vi "test_scope.vi"() -> ()   [LabVIEW 2009]
uses:
  <instrlib>/Agilent 8000 Series/Agilent 8000 Series.lvlib
panel:
  out "bucle time":u32
  in  "stop while":bool
  in  "Boolean ini":bool
  in  "write buffer ini":string
  in  "byte count 2":u32
  out "return count 4":u32
  out "return count 3":u32
  out "return count 2":u32
  out "return count":u32
  in  "byte count":u32
  out "Numeric":i32
  out "read buffer":string
  out "error out":errorcluster
  in  "VISA resource name":refnum<visa-resource-name>
  in  "stop":bool
  in  "write buffer":string
  out "x-y":u32
  in  "Boolean":bool
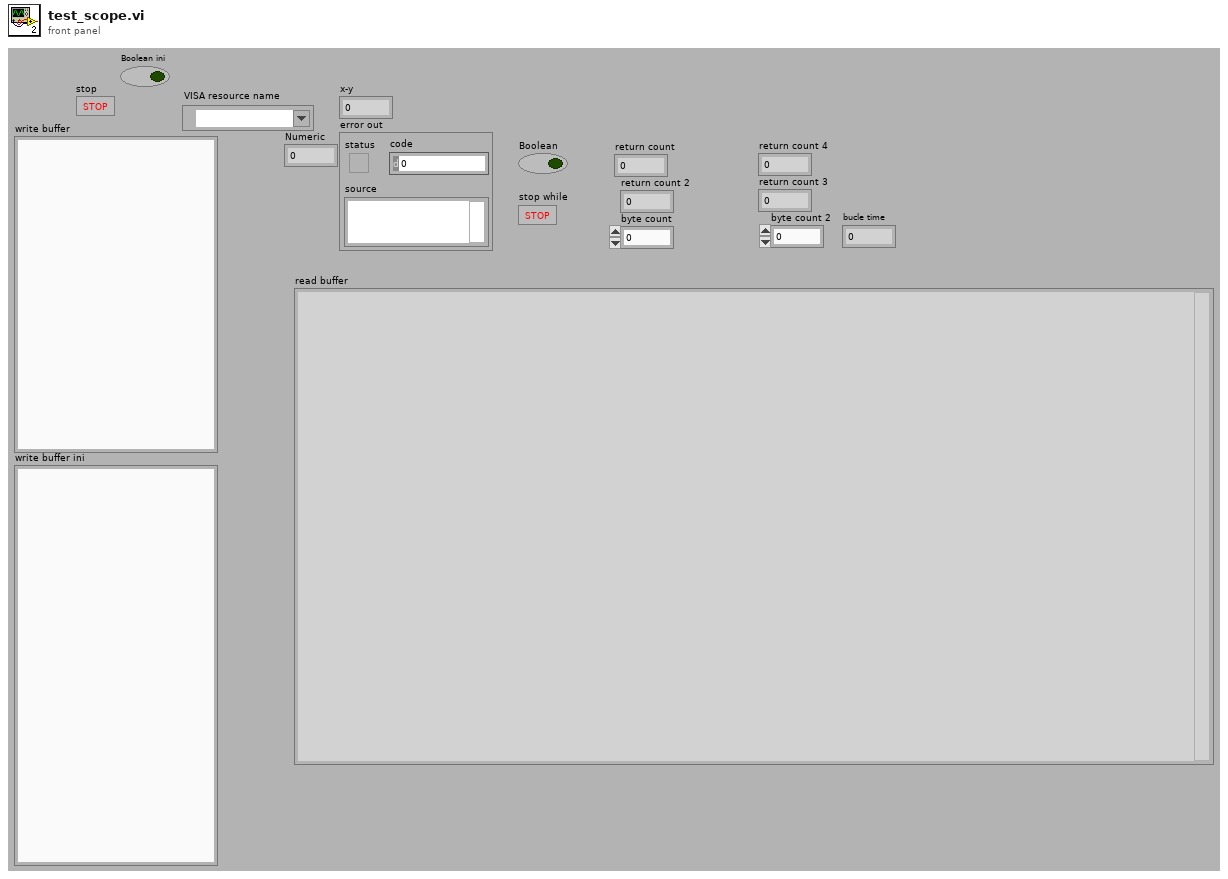
[diagram p1: front panel]
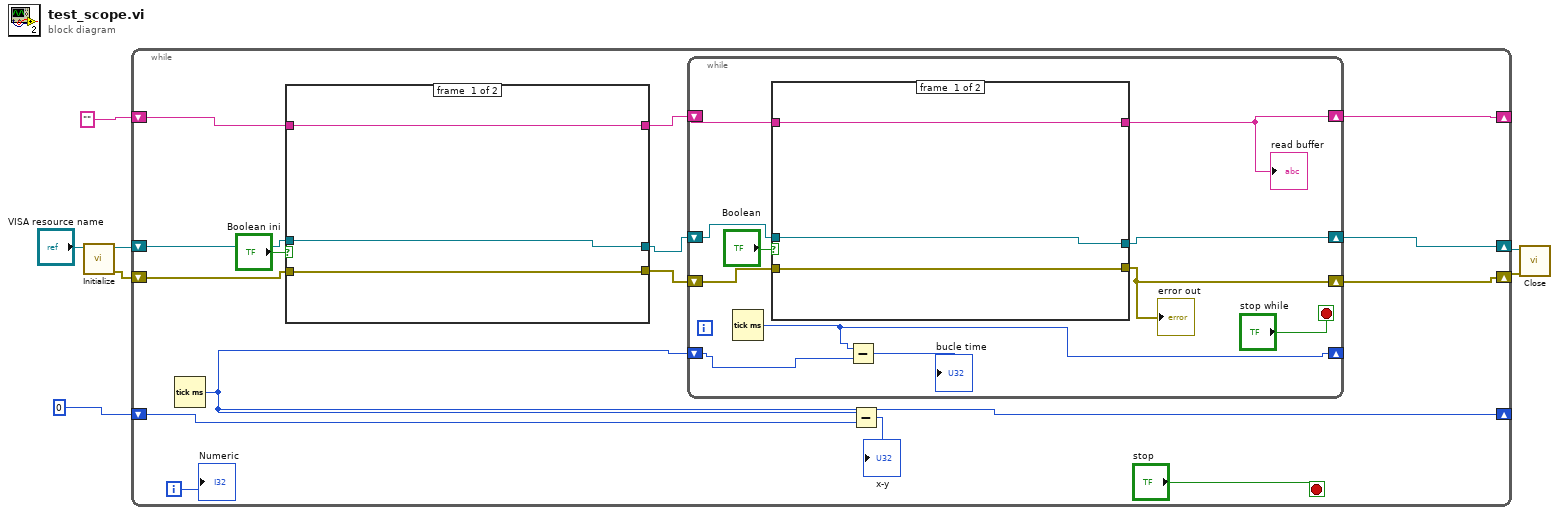
[diagram p0: block diagram]
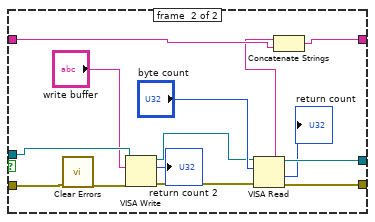
[diagram p2: hidden frame]
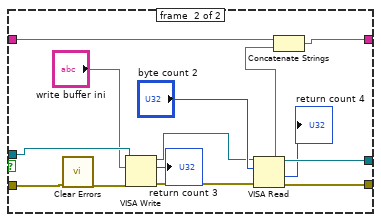
[diagram p3: hidden frame]
diagram:
  n1 = call <instrlib>:"Initialize.vi"("VISA resource name"="VISA resource name") -> ("error out"=w6:errorcluster, "VISA resource name out"=w7:refnum<visa-resource-name>)  [unwired: 9 in]
  n2 = while {
    shift-right: [w8] -> _
    shift-left: u32 0 ("millisecond timer value") -> [w20]
    shift-right: [w22] -> w5
    shift-left: w7 -> [w13]
    shift-right: [w21] -> w4
    shift-left: w6 -> [w15]
    shift-right: [w16] -> _
    shift-left: "" -> [w11]
    i -> [w17]
    stop <- "stop" stop-if-true
    n3 = Tick Count (ms)() -> (millisecond timer value=w8:u32)
    n4 = case shown="True" "Boolean ini" {
      tunnel: w13 -> [w53 w64]
      tunnel: w15 -> [w52 w59]
      tunnel: [w53 w66] -> w9
      tunnel: [w52 w65] -> w14
      tunnel: w11 -> [w51 w62]
      tunnel: [w51 w60] -> w12
      frame #0 {
      }
      frame #1 {
        n5 = call <vilib>:"Clear Errors.vi"("error in (no error)"=w59) -> ("error out"=w58:errorcluster)  [unwired: 6 in]
        n6 = VISA Write(VISA resource name=w64, write buffer="write buffer ini", error in (no error)=w58) -> (VISA resource name out=w56:refnum<visa-resource-name>, return count=→"return count 3":u32, error out=w67:errorcluster)
        n7 = VISA Read(VISA resource name=w56, byte count="byte count 2", error in (no error)=w67) -> (VISA resource name out=w66:refnum<visa-resource-name>, read buffer=w61:string, return count=→"return count 4":u32, error out=w65:errorcluster)
        n8 = Concatenate Strings(w62, w61) -> (w60:string)
      }
    }
    n9 = while {
      shift-right: [w30] -> w16
      shift-left: w12 -> [w28]
      shift-right: [w33] -> w22
      shift-left: w9 -> [w26]
      shift-right: [w32] -> w21
      shift-left: w14 -> [w29]
      shift-right: [w23] -> _
      shift-left: w8 -> [w24]
      stop <- "stop while" stop-if-true
      n10 = Tick Count (ms)() -> (millisecond timer value=w23:u32)
      n11 = case shown="True" "Boolean" {
        tunnel: w26 -> [w36 w47]
        tunnel: w29 -> [w35 w44]
        tunnel: [w36 w49] -> w33
        tunnel: [w35 w48] -> w32
        tunnel: w28 -> [w34 w38]
        tunnel: [w34 w45] -> w30
        frame #0 {
        }
        frame #1 {
          n12 = call <vilib>:"Clear Errors.vi"("error in (no error)"=w44) -> ("error out"=w43:errorcluster)  [unwired: 6 in]
          n13 = VISA Write(VISA resource name=w47, write buffer="write buffer", error in (no error)=w43) -> (VISA resource name out=w41:refnum<visa-resource-name>, return count=→"return count 2":u32, error out=w50:errorcluster)
          n14 = VISA Read(VISA resource name=w41, byte count="byte count", error in (no error)=w50) -> (VISA resource name out=w49:refnum<visa-resource-name>, read buffer=w37:string, return count=→"return count":u32, error out=w48:errorcluster)
          n15 = Concatenate Strings(w37, w38) -> (w45:string)
        }
      }
      "error out" <- w32
      "read buffer" <- w30
      n16 = Subtract(x=w23, y=w24) -> (x-y=→"bucle time":u32)
    }
    n17 = Subtract(x=w8, y=w20) -> (x-y=→"x-y":u32)
    "Numeric" <- w17
  }
  n18 = call <instrlib>:"Close.vi"("error in (no error)"=w4, "VISA resource name"=w5) -> ()  [unwired: 9 in, 1 out]
